vi "RegisterEvent.vi"(8 "error in (no error)":errorcluster, 9 "EventDataUserEvent":refnum<user-event>, 10 "EventData":refnum<class "EventData.lvclass">, 11 "EventManager in":refnum<class "EventManager.lvclass">) -> (0 "error out":errorcluster, 1 "EventToken":refnum<class "EventToken.lvclass">, 3 "EventManager out":refnum<class "EventManager.lvclass">)   [LabVIEW 2009, in "EventManagerLibrary.lvlib" / "EventManager.lvclass"]
uses:
  EventManager.lvclass
  EventDataObject/EventData.lvclass
  EventToken/EventToken.lvclass
  EventObject/Event.lvclass
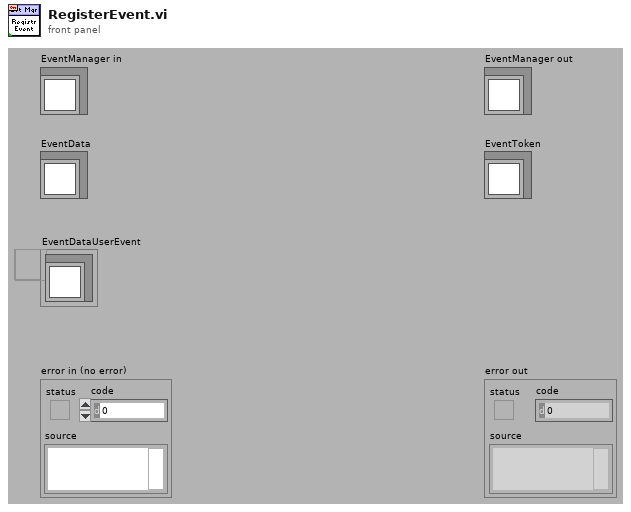
[diagram p1: front panel]
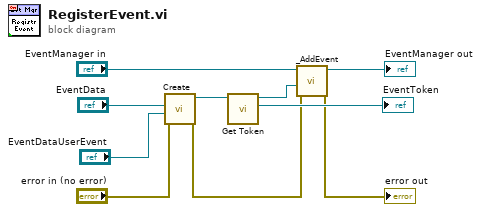
[diagram p0: block diagram]
diagram:
  n1 = call "Create.vi"("error in (no error)"="error in (no error)", "EventDataUserEvent"="EventDataUserEvent", "EventData"="EventData") -> ("error out"=w2:errorcluster, "Event out"=w5:refnum<class "Event.lvclass">)  [unwired: 7 out]
  n2 = call-dynamic "Get Token.vi"("Event in"=w5) -> ("EventToken"=→"EventToken":refnum<class "EventToken.lvclass">, "Event out"=w3:refnum<class "Event.lvclass">)  [unwired: 1 in, 8 out]
  n3 = call "_AddEvent.vi"("error in (no error)"=w2, "Event"=w3, "EventManager in"="EventManager in") -> ("error out"=→"error out":errorcluster, "EventManager out"=→"EventManager out":refnum<class "EventManager.lvclass">)  [unwired: 7 out]
